vi "Convert String.vi"(4 "dst byte order":T3(ring), 5 "src channel descriptor":T1 {"buffer offset" format="%d bytes"}, 6 "src byte order":T3(ring), 7 "dst channel descriptor":T1 {"buffer offset" format="%d bytes"}, 8 "error in (no error)":errorcluster, 9 "channel count":u64, 10 "dst buffer in":string, 11 "src buffer in":string) -> (0 "error out":errorcluster, 2 "dst buffer out":string, 3 "src buffer out":string)   [LabVIEW 2017, in "DSF Core.lvlib" / "Buffer Converter.lvclass"]
uses:
  Buffer Converter.lvclass
  Block Descriptor.ctl
  DSF Configuration API/Public/Controls/DSF Data Type.ctl
  Shared/VIs/Sizeof.vi
  DSF Core.lvlib
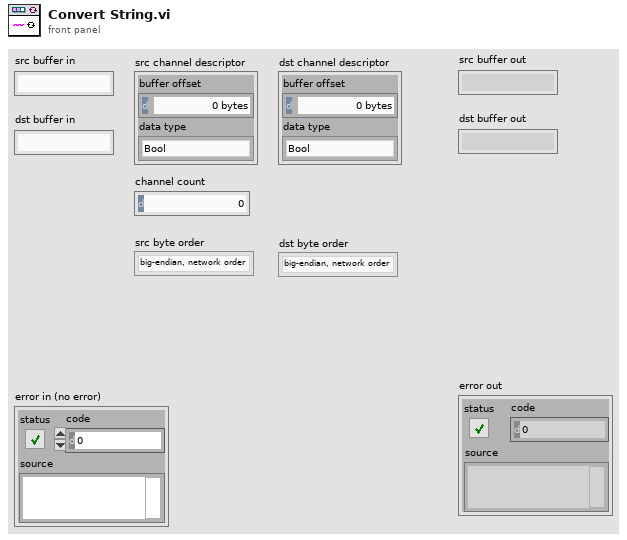
[diagram p1: front panel]
types:
  T1 = typedef "DSF Core.lvlib/Buffer Converter.lvclass/Block Descriptor.ctl" = cluster{"buffer offset":u64, "data type":T2}
  T2 = typedef "DSF Core.lvlib/DSF Data Type.ctl" = enum8{"Bool", "SGL", "DBL", "I8", "I16", "I32", "I64", "U8", "U16", "U32", "U64"}
  T3 = enum16{"big-endian, network order", "native, host order", "little-endian"}
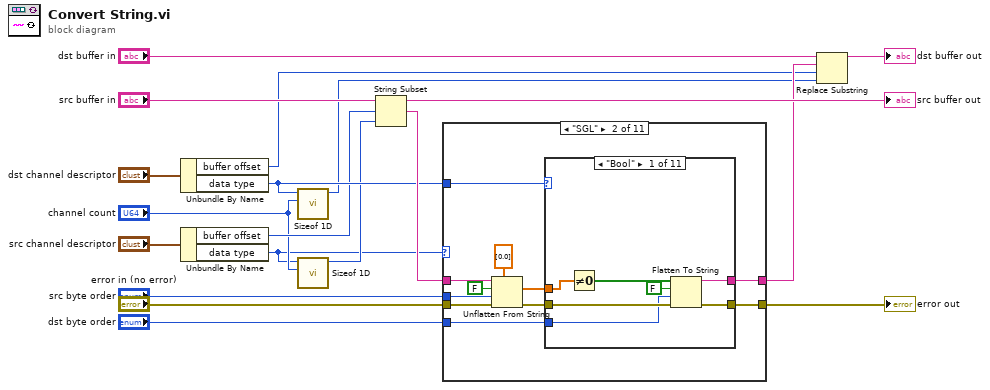
[diagram p0: block diagram]
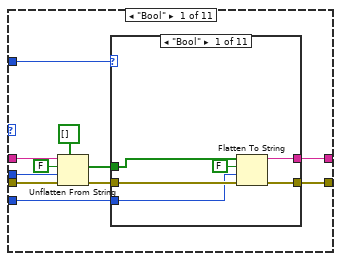
[diagram p2: hidden frame]
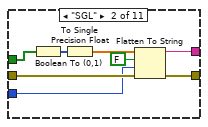
[diagram p3: hidden frame]
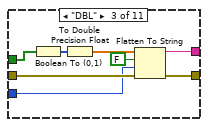
[diagram p4: hidden frame]
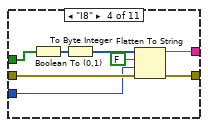
[diagram p5: hidden frame]
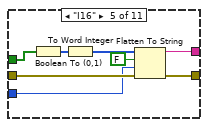
[diagram p6: hidden frame]
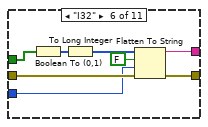
[diagram p7: hidden frame]
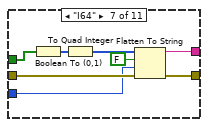
[diagram p8: hidden frame]
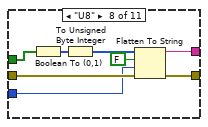
[diagram p9: hidden frame]
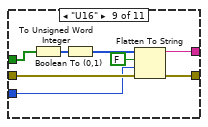
[diagram p10: hidden frame]
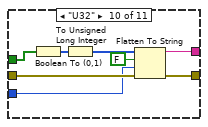
[diagram p11: hidden frame]
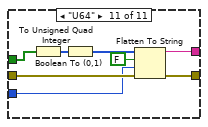
[diagram p12: hidden frame]
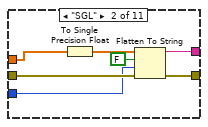
[diagram p13: hidden frame]
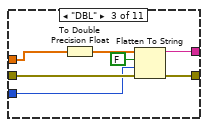
[diagram p14: hidden frame]
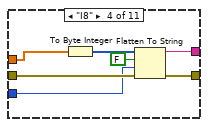
[diagram p15: hidden frame]
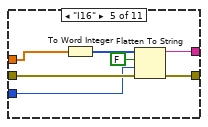
[diagram p16: hidden frame]
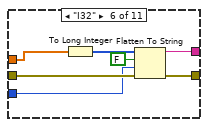
[diagram p17: hidden frame]
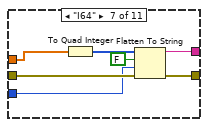
[diagram p18: hidden frame]
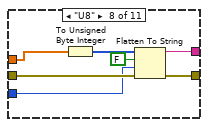
[diagram p19: hidden frame]
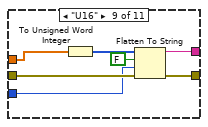
[diagram p20: hidden frame]
diagram:
  n1 = Unbundle By Name("dst channel descriptor") -> ("buffer offset"=w1:u64, "data type"=w10:T2)
  n2 = Unbundle By Name("src channel descriptor") -> ("buffer offset"=w9:u64, "data type"=w4:T2)
  n3 = call "Sizeof 1D.vi"("count"="channel count", "data type"=w10) -> ("size in bytes"=w2:u64)  [unwired: 9 in]
  n4 = call "Sizeof 1D.vi"("count"="channel count", "data type"=w4) -> ("size in bytes"=w8:u64)  [unwired: 9 in]
  n5 = String Subset(string="src buffer in", offset (0)=w9, length (rest)=w8) -> (substring=w11:string)
  n6 = case shown="\"SGL\"" w4 {
    tunnel: w11 -> [w27 w124 w212 w300 w388 w476 w564 w652 w740 w828 w916]
    tunnel: "error in (no error)" -> [w26 w123 w211 w299 w387 w475 w563 w651 w739 w827 w915]
    tunnel: w10 -> [w25 w122 w210 w298 w386 w474 w562 w650 w738 w826 w914]
    tunnel: [w22 w119 w207 w295 w383 w471 w559 w647 w735 w823 w911] -> w16
    tunnel: [w21 w118 w206 w294 w382 w470 w558 w646 w734 w822 w910] -> w3
    tunnel: "src byte order" -> [w20 w117 w205 w293 w381 w469 w557 w645 w733 w821 w909]
    tunnel: "dst byte order" -> [w19 w116 w204 w292 w380 w468 w556 w644 w732 w820 w908]
    frame "Bool" {
      n7 = Unflatten From String(type=bool[] [], binary string=w27, data includes array or string size? (T)=FALSE, byte order (0:big-endian, network order)=w20, error in (no error)=w26) -> (value=w24:bool[], error out=w23:errorcluster)  [unwired: 1 out]
      n8 = case shown="\"Bool\"" w25 {
        tunnel: w24 -> [w35 w43 w51 w59 w67 w75 w83 w91 w99 w107 w115]
        tunnel: w23 -> [w34 w42 w50 w58 w66 w74 w82 w90 w98 w106 w114]
        tunnel: [w33 w41 w49 w57 w65 w73 w81 w89 w97 w105 w113] -> w22
        tunnel: [w32 w40 w48 w56 w64 w72 w80 w88 w96 w104 w112] -> w21
        tunnel: w19 -> [w31 w39 w47 w55 w63 w71 w79 w87 w95 w103 w111]
        frame "Bool" {
          n9 = Flatten To String(anything=w35, prepend array or string size? (T)=FALSE, byte order (0:big-endian, network order)=w31, error in (no error)=w34) -> (data string=w32:string, error out=w33:errorcluster)  [unwired: 1 out]
        }
        frame "SGL" {
          n10 = Boolean To (0,1)(Boolean=w43) -> (0, 1=w36:i16[])
          n11 = To Single Precision Float(number=w36) -> (single precision float=w37:sgl[])
          n12 = Flatten To String(anything=w37, prepend array or string size? (T)=FALSE, byte order (0:big-endian, network order)=w39, error in (no error)=w42) -> (data string=w40:string, error out=w41:errorcluster)  [unwired: 1 out]
        }
        frame "DBL" {
          n13 = Boolean To (0,1)(Boolean=w51) -> (0, 1=w44:i16[])
          n14 = To Double Precision Float(number=w44) -> (double precision float=w45:dbl[])
          n15 = Flatten To String(anything=w45, prepend array or string size? (T)=FALSE, byte order (0:big-endian, network order)=w47, error in (no error)=w50) -> (data string=w48:string, error out=w49:errorcluster)  [unwired: 1 out]
        }
        frame "I8" {
          n16 = Boolean To (0,1)(Boolean=w59) -> (0, 1=w52:i16[])
          n17 = To Byte Integer(number=w52) -> (8bit integer=w53:i8[])
          n18 = Flatten To String(anything=w53, prepend array or string size? (T)=FALSE, byte order (0:big-endian, network order)=w55, error in (no error)=w58) -> (data string=w56:string, error out=w57:errorcluster)  [unwired: 1 out]
        }
        frame "I16" {
          n19 = Boolean To (0,1)(Boolean=w67) -> (0, 1=w60:i16[])
          n20 = To Word Integer(number=w60) -> (16bit integer=w61:i16[])
          n21 = Flatten To String(anything=w61, prepend array or string size? (T)=FALSE, byte order (0:big-endian, network order)=w63, error in (no error)=w66) -> (data string=w64:string, error out=w65:errorcluster)  [unwired: 1 out]
        }
        frame "I32" {
          n22 = Boolean To (0,1)(Boolean=w75) -> (0, 1=w68:i16[])
          n23 = To Long Integer(number=w68) -> (32bit integer=w69:i32[])
          n24 = Flatten To String(anything=w69, prepend array or string size? (T)=FALSE, byte order (0:big-endian, network order)=w71, error in (no error)=w74) -> (data string=w72:string, error out=w73:errorcluster)  [unwired: 1 out]
        }
        frame "I64" {
          n25 = Boolean To (0,1)(Boolean=w83) -> (0, 1=w76:i16[])
          n26 = To Quad Integer(1:w76) -> (0:w77:i64[])
          n27 = Flatten To String(anything=w77, prepend array or string size? (T)=FALSE, byte order (0:big-endian, network order)=w79, error in (no error)=w82) -> (data string=w80:string, error out=w81:errorcluster)  [unwired: 1 out]
        }
        frame "U8" {
          n28 = Boolean To (0,1)(Boolean=w91) -> (0, 1=w84:i16[])
          n29 = To Unsigned Byte Integer(number=w84) -> (unsigned 8bit integer=w85:u8[])
          n30 = Flatten To String(anything=w85, prepend array or string size? (T)=FALSE, byte order (0:big-endian, network order)=w87, error in (no error)=w90) -> (data string=w88:string, error out=w89:errorcluster)  [unwired: 1 out]
        }
        frame "U16" {
          n31 = Boolean To (0,1)(Boolean=w99) -> (0, 1=w92:i16[])
          n32 = To Unsigned Word Integer(number=w92) -> (unsigned 16bit integer=w93:u16[])
          n33 = Flatten To String(anything=w93, prepend array or string size? (T)=FALSE, byte order (0:big-endian, network order)=w95, error in (no error)=w98) -> (data string=w96:string, error out=w97:errorcluster)  [unwired: 1 out]
        }
        frame "U32" {
          n34 = Boolean To (0,1)(Boolean=w107) -> (0, 1=w100:i16[])
          n35 = To Unsigned Long Integer(number=w100) -> (unsigned 32bit integer=w101:u32[])
          n36 = Flatten To String(anything=w101, prepend array or string size? (T)=FALSE, byte order (0:big-endian, network order)=w103, error in (no error)=w106) -> (data string=w104:string, error out=w105:errorcluster)  [unwired: 1 out]
        }
        frame "U64" {
          n37 = Boolean To (0,1)(Boolean=w115) -> (0, 1=w108:i16[])
          n38 = To Unsigned Quad Integer(1:w108) -> (0:w109:u64[])
          n39 = Flatten To String(anything=w109, prepend array or string size? (T)=FALSE, byte order (0:big-endian, network order)=w111, error in (no error)=w114) -> (data string=w112:string, error out=w113:errorcluster)  [unwired: 1 out]
        }
      }
    }
    frame "SGL" {
      n40 = Unflatten From String(type=sgl[] [0.0], binary string=w124, data includes array or string size? (T)=FALSE, byte order (0:big-endian, network order)=w117, error in (no error)=w123) -> (value=w121:sgl[], error out=w120:errorcluster)  [unwired: 1 out]
      n41 = case shown="\"Bool\"" w122 {
        tunnel: w121 -> [w128 w135 w142 w149 w156 w163 w170 w177 w184 w191 w198]
        tunnel: w120 -> [w133 w140 w147 w154 w161 w168 w175 w182 w189 w196 w203]
        tunnel: [w132 w139 w146 w153 w160 w167 w174 w181 w188 w195 w202] -> w119
        tunnel: [w131 w138 w145 w152 w159 w166 w173 w180 w187 w194 w201] -> w118
        tunnel: w116 -> [w130 w137 w144 w151 w158 w165 w172 w179 w186 w193 w200]
        frame "Bool" {
          n42 = Not Equal To 0?(x=w128) -> (x != 0?=w127:bool[])
          n43 = Flatten To String(anything=w127, prepend array or string size? (T)=FALSE, byte order (0:big-endian, network order)=w130, error in (no error)=w133) -> (data string=w131:string, error out=w132:errorcluster)  [unwired: 1 out]
        }
        frame "SGL" {
          n44 = To Single Precision Float(number=w135) -> (single precision float=w134:sgl[])
          n45 = Flatten To String(anything=w134, prepend array or string size? (T)=FALSE, byte order (0:big-endian, network order)=w137, error in (no error)=w140) -> (data string=w138:string, error out=w139:errorcluster)  [unwired: 1 out]
        }
        frame "DBL" {
          n46 = To Double Precision Float(number=w142) -> (double precision float=w141:dbl[])
          n47 = Flatten To String(anything=w141, prepend array or string size? (T)=FALSE, byte order (0:big-endian, network order)=w144, error in (no error)=w147) -> (data string=w145:string, error out=w146:errorcluster)  [unwired: 1 out]
        }
        frame "I8" {
          n48 = To Byte Integer(number=w149) -> (8bit integer=w148:i8[])
          n49 = Flatten To String(anything=w148, prepend array or string size? (T)=FALSE, byte order (0:big-endian, network order)=w151, error in (no error)=w154) -> (data string=w152:string, error out=w153:errorcluster)  [unwired: 1 out]
        }
        frame "I16" {
          n50 = To Word Integer(number=w156) -> (16bit integer=w155:i16[])
          n51 = Flatten To String(anything=w155, prepend array or string size? (T)=FALSE, byte order (0:big-endian, network order)=w158, error in (no error)=w161) -> (data string=w159:string, error out=w160:errorcluster)  [unwired: 1 out]
        }
        frame "I32" {
          n52 = To Long Integer(number=w163) -> (32bit integer=w162:i32[])
          n53 = Flatten To String(anything=w162, prepend array or string size? (T)=FALSE, byte order (0:big-endian, network order)=w165, error in (no error)=w168) -> (data string=w166:string, error out=w167:errorcluster)  [unwired: 1 out]
        }
        frame "I64" {
          n54 = To Quad Integer(1:w170) -> (0:w169:i64[])
          n55 = Flatten To String(anything=w169, prepend array or string size? (T)=FALSE, byte order (0:big-endian, network order)=w172, error in (no error)=w175) -> (data string=w173:string, error out=w174:errorcluster)  [unwired: 1 out]
        }
        frame "U8" {
          n56 = To Unsigned Byte Integer(number=w177) -> (unsigned 8bit integer=w176:u8[])
          n57 = Flatten To String(anything=w176, prepend array or string size? (T)=FALSE, byte order (0:big-endian, network order)=w179, error in (no error)=w182) -> (data string=w180:string, error out=w181:errorcluster)  [unwired: 1 out]
        }
        frame "U16" {
          n58 = To Unsigned Word Integer(number=w184) -> (unsigned 16bit integer=w183:u16[])
          n59 = Flatten To String(anything=w183, prepend array or string size? (T)=FALSE, byte order (0:big-endian, network order)=w186, error in (no error)=w189) -> (data string=w187:string, error out=w188:errorcluster)  [unwired: 1 out]
        }
        frame "U32" {
          n60 = To Unsigned Long Integer(number=w191) -> (unsigned 32bit integer=w190:u32[])
          n61 = Flatten To String(anything=w190, prepend array or string size? (T)=FALSE, byte order (0:big-endian, network order)=w193, error in (no error)=w196) -> (data string=w194:string, error out=w195:errorcluster)  [unwired: 1 out]
        }
        frame "U64" {
          n62 = To Unsigned Quad Integer(1:w198) -> (0:w197:u64[])
          n63 = Flatten To String(anything=w197, prepend array or string size? (T)=FALSE, byte order (0:big-endian, network order)=w200, error in (no error)=w203) -> (data string=w201:string, error out=w202:errorcluster)  [unwired: 1 out]
        }
      }
    }
    frame "DBL" {
      n64 = Unflatten From String(type=dbl[] [0.0], binary string=w212, data includes array or string size? (T)=FALSE, byte order (0:big-endian, network order)=w205, error in (no error)=w211) -> (value=w209:dbl[], error out=w208:errorcluster)  [unwired: 1 out]
      n65 = case shown="\"I8\"" w210 {
        tunnel: w209 -> [w216 w223 w230 w237 w244 w251 w258 w265 w272 w279 w286]
        tunnel: w208 -> [w221 w228 w235 w242 w249 w256 w263 w270 w277 w284 w291]
        tunnel: [w220 w227 w234 w241 w248 w255 w262 w269 w276 w283 w290] -> w207
        tunnel: [w219 w226 w233 w240 w247 w254 w261 w268 w275 w282 w289] -> w206
        tunnel: w204 -> [w218 w225 w232 w239 w246 w253 w260 w267 w274 w281 w288]
        frame "Bool" {
          n66 = Not Equal To 0?(x=w216) -> (x != 0?=w215:bool[])
          n67 = Flatten To String(anything=w215, prepend array or string size? (T)=FALSE, byte order (0:big-endian, network order)=w218, error in (no error)=w221) -> (data string=w219:string, error out=w220:errorcluster)  [unwired: 1 out]
        }
        frame "SGL" {
          n68 = To Single Precision Float(number=w223) -> (single precision float=w222:sgl[])
          n69 = Flatten To String(anything=w222, prepend array or string size? (T)=FALSE, byte order (0:big-endian, network order)=w225, error in (no error)=w228) -> (data string=w226:string, error out=w227:errorcluster)  [unwired: 1 out]
        }
        frame "DBL" {
          n70 = To Double Precision Float(number=w230) -> (double precision float=w229:dbl[])
          n71 = Flatten To String(anything=w229, prepend array or string size? (T)=FALSE, byte order (0:big-endian, network order)=w232, error in (no error)=w235) -> (data string=w233:string, error out=w234:errorcluster)  [unwired: 1 out]
        }
        frame "I8" {
          n72 = To Byte Integer(number=w237) -> (8bit integer=w236:i8[])
          n73 = Flatten To String(anything=w236, prepend array or string size? (T)=FALSE, byte order (0:big-endian, network order)=w239, error in (no error)=w242) -> (data string=w240:string, error out=w241:errorcluster)  [unwired: 1 out]
        }
        frame "I16" {
          n74 = To Word Integer(number=w244) -> (16bit integer=w243:i16[])
          n75 = Flatten To String(anything=w243, prepend array or string size? (T)=FALSE, byte order (0:big-endian, network order)=w246, error in (no error)=w249) -> (data string=w247:string, error out=w248:errorcluster)  [unwired: 1 out]
        }
        frame "I32" {
          n76 = To Long Integer(number=w251) -> (32bit integer=w250:i32[])
          n77 = Flatten To String(anything=w250, prepend array or string size? (T)=FALSE, byte order (0:big-endian, network order)=w253, error in (no error)=w256) -> (data string=w254:string, error out=w255:errorcluster)  [unwired: 1 out]
        }
        frame "I64" {
          n78 = To Quad Integer(1:w258) -> (0:w257:i64[])
          n79 = Flatten To String(anything=w257, prepend array or string size? (T)=FALSE, byte order (0:big-endian, network order)=w260, error in (no error)=w263) -> (data string=w261:string, error out=w262:errorcluster)  [unwired: 1 out]
        }
        frame "U8" {
          n80 = To Unsigned Byte Integer(number=w265) -> (unsigned 8bit integer=w264:u8[])
          n81 = Flatten To String(anything=w264, prepend array or string size? (T)=FALSE, byte order (0:big-endian, network order)=w267, error in (no error)=w270) -> (data string=w268:string, error out=w269:errorcluster)  [unwired: 1 out]
        }
        frame "U16" {
          n82 = To Unsigned Word Integer(number=w272) -> (unsigned 16bit integer=w271:u16[])
          n83 = Flatten To String(anything=w271, prepend array or string size? (T)=FALSE, byte order (0:big-endian, network order)=w274, error in (no error)=w277) -> (data string=w275:string, error out=w276:errorcluster)  [unwired: 1 out]
        }
        frame "U32" {
          n84 = To Unsigned Long Integer(number=w279) -> (unsigned 32bit integer=w278:u32[])
          n85 = Flatten To String(anything=w278, prepend array or string size? (T)=FALSE, byte order (0:big-endian, network order)=w281, error in (no error)=w284) -> (data string=w282:string, error out=w283:errorcluster)  [unwired: 1 out]
        }
        frame "U64" {
          n86 = To Unsigned Quad Integer(1:w286) -> (0:w285:u64[])
          n87 = Flatten To String(anything=w285, prepend array or string size? (T)=FALSE, byte order (0:big-endian, network order)=w288, error in (no error)=w291) -> (data string=w289:string, error out=w290:errorcluster)  [unwired: 1 out]
        }
      }
    }
    frame "I8" {
      n88 = Unflatten From String(type=i8[] [0], binary string=w300, data includes array or string size? (T)=FALSE, byte order (0:big-endian, network order)=w293, error in (no error)=w299) -> (value=w297:i8[], error out=w296:errorcluster)  [unwired: 1 out]
      n89 = case shown="\"Bool\"" w298 {
        tunnel: w297 -> [w304 w311 w318 w325 w332 w339 w346 w353 w360 w367 w374]
        tunnel: w296 -> [w309 w316 w323 w330 w337 w344 w351 w358 w365 w372 w379]
        tunnel: [w308 w315 w322 w329 w336 w343 w350 w357 w364 w371 w378] -> w295
        tunnel: [w307 w314 w321 w328 w335 w342 w349 w356 w363 w370 w377] -> w294
        tunnel: w292 -> [w306 w313 w320 w327 w334 w341 w348 w355 w362 w369 w376]
        frame "Bool" {
          n90 = Not Equal To 0?(x=w304) -> (x != 0?=w303:bool[])
          n91 = Flatten To String(anything=w303, prepend array or string size? (T)=FALSE, byte order (0:big-endian, network order)=w306, error in (no error)=w309) -> (data string=w307:string, error out=w308:errorcluster)  [unwired: 1 out]
        }
        frame "SGL" {
          n92 = To Single Precision Float(number=w311) -> (single precision float=w310:sgl[])
          n93 = Flatten To String(anything=w310, prepend array or string size? (T)=FALSE, byte order (0:big-endian, network order)=w313, error in (no error)=w316) -> (data string=w314:string, error out=w315:errorcluster)  [unwired: 1 out]
        }
        frame "DBL" {
          n94 = To Double Precision Float(number=w318) -> (double precision float=w317:dbl[])
          n95 = Flatten To String(anything=w317, prepend array or string size? (T)=FALSE, byte order (0:big-endian, network order)=w320, error in (no error)=w323) -> (data string=w321:string, error out=w322:errorcluster)  [unwired: 1 out]
        }
        frame "I8" {
          n96 = To Byte Integer(number=w325) -> (8bit integer=w324:i8[])
          n97 = Flatten To String(anything=w324, prepend array or string size? (T)=FALSE, byte order (0:big-endian, network order)=w327, error in (no error)=w330) -> (data string=w328:string, error out=w329:errorcluster)  [unwired: 1 out]
        }
        frame "I16" {
          n98 = To Word Integer(number=w332) -> (16bit integer=w331:i16[])
          n99 = Flatten To String(anything=w331, prepend array or string size? (T)=FALSE, byte order (0:big-endian, network order)=w334, error in (no error)=w337) -> (data string=w335:string, error out=w336:errorcluster)  [unwired: 1 out]
        }
        frame "I32" {
          n100 = To Long Integer(number=w339) -> (32bit integer=w338:i32[])
          n101 = Flatten To String(anything=w338, prepend array or string size? (T)=FALSE, byte order (0:big-endian, network order)=w341, error in (no error)=w344) -> (data string=w342:string, error out=w343:errorcluster)  [unwired: 1 out]
        }
        frame "I64" {
          n102 = To Quad Integer(1:w346) -> (0:w345:i64[])
          n103 = Flatten To String(anything=w345, prepend array or string size? (T)=FALSE, byte order (0:big-endian, network order)=w348, error in (no error)=w351) -> (data string=w349:string, error out=w350:errorcluster)  [unwired: 1 out]
        }
        frame "U8" {
          n104 = To Unsigned Byte Integer(number=w353) -> (unsigned 8bit integer=w352:u8[])
          n105 = Flatten To String(anything=w352, prepend array or string size? (T)=FALSE, byte order (0:big-endian, network order)=w355, error in (no error)=w358) -> (data string=w356:string, error out=w357:errorcluster)  [unwired: 1 out]
        }
        frame "U16" {
          n106 = To Unsigned Word Integer(number=w360) -> (unsigned 16bit integer=w359:u16[])
          n107 = Flatten To String(anything=w359, prepend array or string size? (T)=FALSE, byte order (0:big-endian, network order)=w362, error in (no error)=w365) -> (data string=w363:string, error out=w364:errorcluster)  [unwired: 1 out]
        }
        frame "U32" {
          n108 = To Unsigned Long Integer(number=w367) -> (unsigned 32bit integer=w366:u32[])
          n109 = Flatten To String(anything=w366, prepend array or string size? (T)=FALSE, byte order (0:big-endian, network order)=w369, error in (no error)=w372) -> (data string=w370:string, error out=w371:errorcluster)  [unwired: 1 out]
        }
        frame "U64" {
          n110 = To Unsigned Quad Integer(1:w374) -> (0:w373:u64[])
          n111 = Flatten To String(anything=w373, prepend array or string size? (T)=FALSE, byte order (0:big-endian, network order)=w376, error in (no error)=w379) -> (data string=w377:string, error out=w378:errorcluster)  [unwired: 1 out]
        }
      }
    }
    frame "I16" {
      n112 = Unflatten From String(type=i16[] [0], binary string=w388, data includes array or string size? (T)=FALSE, byte order (0:big-endian, network order)=w381, error in (no error)=w387) -> (value=w385:i16[], error out=w384:errorcluster)  [unwired: 1 out]
      n113 = case shown="\"Bool\"" w386 {
        tunnel: w385 -> [w392 w399 w406 w413 w420 w427 w434 w441 w448 w455 w462]
        tunnel: w384 -> [w397 w404 w411 w418 w425 w432 w439 w446 w453 w460 w467]
        tunnel: [w396 w403 w410 w417 w424 w431 w438 w445 w452 w459 w466] -> w383
        tunnel: [w395 w402 w409 w416 w423 w430 w437 w444 w451 w458 w465] -> w382
        tunnel: w380 -> [w394 w401 w408 w415 w422 w429 w436 w443 w450 w457 w464]
        frame "Bool" {
          n114 = Not Equal To 0?(x=w392) -> (x != 0?=w391:bool[])
          n115 = Flatten To String(anything=w391, prepend array or string size? (T)=FALSE, byte order (0:big-endian, network order)=w394, error in (no error)=w397) -> (data string=w395:string, error out=w396:errorcluster)  [unwired: 1 out]
        }
        frame "SGL" {
          n116 = To Single Precision Float(number=w399) -> (single precision float=w398:sgl[])
          n117 = Flatten To String(anything=w398, prepend array or string size? (T)=FALSE, byte order (0:big-endian, network order)=w401, error in (no error)=w404) -> (data string=w402:string, error out=w403:errorcluster)  [unwired: 1 out]
        }
        frame "DBL" {
          n118 = To Double Precision Float(number=w406) -> (double precision float=w405:dbl[])
          n119 = Flatten To String(anything=w405, prepend array or string size? (T)=FALSE, byte order (0:big-endian, network order)=w408, error in (no error)=w411) -> (data string=w409:string, error out=w410:errorcluster)  [unwired: 1 out]
        }
        frame "I8" {
          n120 = To Byte Integer(number=w413) -> (8bit integer=w412:i8[])
          n121 = Flatten To String(anything=w412, prepend array or string size? (T)=FALSE, byte order (0:big-endian, network order)=w415, error in (no error)=w418) -> (data string=w416:string, error out=w417:errorcluster)  [unwired: 1 out]
        }
        frame "I16" {
          n122 = To Word Integer(number=w420) -> (16bit integer=w419:i16[])
          n123 = Flatten To String(anything=w419, prepend array or string size? (T)=FALSE, byte order (0:big-endian, network order)=w422, error in (no error)=w425) -> (data string=w423:string, error out=w424:errorcluster)  [unwired: 1 out]
        }
        frame "I32" {
          n124 = To Long Integer(number=w427) -> (32bit integer=w426:i32[])
          n125 = Flatten To String(anything=w426, prepend array or string size? (T)=FALSE, byte order (0:big-endian, network order)=w429, error in (no error)=w432) -> (data string=w430:string, error out=w431:errorcluster)  [unwired: 1 out]
        }
        frame "I64" {
          n126 = To Quad Integer(1:w434) -> (0:w433:i64[])
          n127 = Flatten To String(anything=w433, prepend array or string size? (T)=FALSE, byte order (0:big-endian, network order)=w436, error in (no error)=w439) -> (data string=w437:string, error out=w438:errorcluster)  [unwired: 1 out]
        }
        frame "U8" {
          n128 = To Unsigned Byte Integer(number=w441) -> (unsigned 8bit integer=w440:u8[])
          n129 = Flatten To String(anything=w440, prepend array or string size? (T)=FALSE, byte order (0:big-endian, network order)=w443, error in (no error)=w446) -> (data string=w444:string, error out=w445:errorcluster)  [unwired: 1 out]
        }
        frame "U16" {
          n130 = To Unsigned Word Integer(number=w448) -> (unsigned 16bit integer=w447:u16[])
          n131 = Flatten To String(anything=w447, prepend array or string size? (T)=FALSE, byte order (0:big-endian, network order)=w450, error in (no error)=w453) -> (data string=w451:string, error out=w452:errorcluster)  [unwired: 1 out]
        }
        frame "U32" {
          n132 = To Unsigned Long Integer(number=w455) -> (unsigned 32bit integer=w454:u32[])
          n133 = Flatten To String(anything=w454, prepend array or string size? (T)=FALSE, byte order (0:big-endian, network order)=w457, error in (no error)=w460) -> (data string=w458:string, error out=w459:errorcluster)  [unwired: 1 out]
        }
        frame "U64" {
          n134 = To Unsigned Quad Integer(1:w462) -> (0:w461:u64[])
          n135 = Flatten To String(anything=w461, prepend array or string size? (T)=FALSE, byte order (0:big-endian, network order)=w464, error in (no error)=w467) -> (data string=w465:string, error out=w466:errorcluster)  [unwired: 1 out]
        }
      }
    }
    frame "I32" {
      n136 = Unflatten From String(type=i32[] [0], binary string=w476, data includes array or string size? (T)=FALSE, byte order (0:big-endian, network order)=w469, error in (no error)=w475) -> (value=w473:i32[], error out=w472:errorcluster)  [unwired: 1 out]
      n137 = case shown="\"Bool\"" w474 {
        tunnel: w473 -> [w480 w487 w494 w501 w508 w515 w522 w529 w536 w543 w550]
        tunnel: w472 -> [w485 w492 w499 w506 w513 w520 w527 w534 w541 w548 w555]
        tunnel: [w484 w491 w498 w505 w512 w519 w526 w533 w540 w547 w554] -> w471
        tunnel: [w483 w490 w497 w504 w511 w518 w525 w532 w539 w546 w553] -> w470
        tunnel: w468 -> [w482 w489 w496 w503 w510 w517 w524 w531 w538 w545 w552]
        frame "Bool" {
          n138 = Not Equal To 0?(x=w480) -> (x != 0?=w479:bool[])
          n139 = Flatten To String(anything=w479, prepend array or string size? (T)=FALSE, byte order (0:big-endian, network order)=w482, error in (no error)=w485) -> (data string=w483:string, error out=w484:errorcluster)  [unwired: 1 out]
        }
        frame "SGL" {
          n140 = To Single Precision Float(number=w487) -> (single precision float=w486:sgl[])
          n141 = Flatten To String(anything=w486, prepend array or string size? (T)=FALSE, byte order (0:big-endian, network order)=w489, error in (no error)=w492) -> (data string=w490:string, error out=w491:errorcluster)  [unwired: 1 out]
        }
        frame "DBL" {
          n142 = To Double Precision Float(number=w494) -> (double precision float=w493:dbl[])
          n143 = Flatten To String(anything=w493, prepend array or string size? (T)=FALSE, byte order (0:big-endian, network order)=w496, error in (no error)=w499) -> (data string=w497:string, error out=w498:errorcluster)  [unwired: 1 out]
        }
        frame "I8" {
          n144 = To Byte Integer(number=w501) -> (8bit integer=w500:i8[])
          n145 = Flatten To String(anything=w500, prepend array or string size? (T)=FALSE, byte order (0:big-endian, network order)=w503, error in (no error)=w506) -> (data string=w504:string, error out=w505:errorcluster)  [unwired: 1 out]
        }
        frame "I16" {
          n146 = To Word Integer(number=w508) -> (16bit integer=w507:i16[])
          n147 = Flatten To String(anything=w507, prepend array or string size? (T)=FALSE, byte order (0:big-endian, network order)=w510, error in (no error)=w513) -> (data string=w511:string, error out=w512:errorcluster)  [unwired: 1 out]
        }
        frame "I32" {
          n148 = To Long Integer(number=w515) -> (32bit integer=w514:i32[])
          n149 = Flatten To String(anything=w514, prepend array or string size? (T)=FALSE, byte order (0:big-endian, network order)=w517, error in (no error)=w520) -> (data string=w518:string, error out=w519:errorcluster)  [unwired: 1 out]
        }
        frame "I64" {
          n150 = To Quad Integer(1:w522) -> (0:w521:i64[])
          n151 = Flatten To String(anything=w521, prepend array or string size? (T)=FALSE, byte order (0:big-endian, network order)=w524, error in (no error)=w527) -> (data string=w525:string, error out=w526:errorcluster)  [unwired: 1 out]
        }
        frame "U8" {
          n152 = To Unsigned Byte Integer(number=w529) -> (unsigned 8bit integer=w528:u8[])
          n153 = Flatten To String(anything=w528, prepend array or string size? (T)=FALSE, byte order (0:big-endian, network order)=w531, error in (no error)=w534) -> (data string=w532:string, error out=w533:errorcluster)  [unwired: 1 out]
        }
        frame "U16" {
          n154 = To Unsigned Word Integer(number=w536) -> (unsigned 16bit integer=w535:u16[])
          n155 = Flatten To String(anything=w535, prepend array or string size? (T)=FALSE, byte order (0:big-endian, network order)=w538, error in (no error)=w541) -> (data string=w539:string, error out=w540:errorcluster)  [unwired: 1 out]
        }
        frame "U32" {
          n156 = To Unsigned Long Integer(number=w543) -> (unsigned 32bit integer=w542:u32[])
          n157 = Flatten To String(anything=w542, prepend array or string size? (T)=FALSE, byte order (0:big-endian, network order)=w545, error in (no error)=w548) -> (data string=w546:string, error out=w547:errorcluster)  [unwired: 1 out]
        }
        frame "U64" {
          n158 = To Unsigned Quad Integer(1:w550) -> (0:w549:u64[])
          n159 = Flatten To String(anything=w549, prepend array or string size? (T)=FALSE, byte order (0:big-endian, network order)=w552, error in (no error)=w555) -> (data string=w553:string, error out=w554:errorcluster)  [unwired: 1 out]
        }
      }
    }
    frame "I64" {
      n160 = Unflatten From String(type=i64[] [0], binary string=w564, data includes array or string size? (T)=FALSE, byte order (0:big-endian, network order)=w557, error in (no error)=w563) -> (value=w561:i64[], error out=w560:errorcluster)  [unwired: 1 out]
      n161 = case shown="\"Bool\"" w562 {
        tunnel: w561 -> [w568 w575 w582 w589 w596 w603 w610 w617 w624 w631 w638]
        tunnel: w560 -> [w573 w580 w587 w594 w601 w608 w615 w622 w629 w636 w643]
        tunnel: [w572 w579 w586 w593 w600 w607 w614 w621 w628 w635 w642] -> w559
        tunnel: [w571 w578 w585 w592 w599 w606 w613 w620 w627 w634 w641] -> w558
        tunnel: w556 -> [w570 w577 w584 w591 w598 w605 w612 w619 w626 w633 w640]
        frame "Bool" {
          n162 = Not Equal To 0?(x=w568) -> (x != 0?=w567:bool[])
          n163 = Flatten To String(anything=w567, prepend array or string size? (T)=FALSE, byte order (0:big-endian, network order)=w570, error in (no error)=w573) -> (data string=w571:string, error out=w572:errorcluster)  [unwired: 1 out]
        }
        frame "SGL" {
          n164 = To Single Precision Float(number=w575) -> (single precision float=w574:sgl[])
          n165 = Flatten To String(anything=w574, prepend array or string size? (T)=FALSE, byte order (0:big-endian, network order)=w577, error in (no error)=w580) -> (data string=w578:string, error out=w579:errorcluster)  [unwired: 1 out]
        }
        frame "DBL" {
          n166 = To Double Precision Float(number=w582) -> (double precision float=w581:dbl[])
          n167 = Flatten To String(anything=w581, prepend array or string size? (T)=FALSE, byte order (0:big-endian, network order)=w584, error in (no error)=w587) -> (data string=w585:string, error out=w586:errorcluster)  [unwired: 1 out]
        }
        frame "I8" {
          n168 = To Byte Integer(number=w589) -> (8bit integer=w588:i8[])
          n169 = Flatten To String(anything=w588, prepend array or string size? (T)=FALSE, byte order (0:big-endian, network order)=w591, error in (no error)=w594) -> (data string=w592:string, error out=w593:errorcluster)  [unwired: 1 out]
        }
        frame "I16" {
          n170 = To Word Integer(number=w596) -> (16bit integer=w595:i16[])
          n171 = Flatten To String(anything=w595, prepend array or string size? (T)=FALSE, byte order (0:big-endian, network order)=w598, error in (no error)=w601) -> (data string=w599:string, error out=w600:errorcluster)  [unwired: 1 out]
        }
        frame "I32" {
          n172 = To Long Integer(number=w603) -> (32bit integer=w602:i32[])
          n173 = Flatten To String(anything=w602, prepend array or string size? (T)=FALSE, byte order (0:big-endian, network order)=w605, error in (no error)=w608) -> (data string=w606:string, error out=w607:errorcluster)  [unwired: 1 out]
        }
        frame "I64" {
          n174 = To Quad Integer(1:w610) -> (0:w609:i64[])
          n175 = Flatten To String(anything=w609, prepend array or string size? (T)=FALSE, byte order (0:big-endian, network order)=w612, error in (no error)=w615) -> (data string=w613:string, error out=w614:errorcluster)  [unwired: 1 out]
        }
        frame "U8" {
          n176 = To Unsigned Byte Integer(number=w617) -> (unsigned 8bit integer=w616:u8[])
          n177 = Flatten To String(anything=w616, prepend array or string size? (T)=FALSE, byte order (0:big-endian, network order)=w619, error in (no error)=w622) -> (data string=w620:string, error out=w621:errorcluster)  [unwired: 1 out]
        }
        frame "U16" {
          n178 = To Unsigned Word Integer(number=w624) -> (unsigned 16bit integer=w623:u16[])
          n179 = Flatten To String(anything=w623, prepend array or string size? (T)=FALSE, byte order (0:big-endian, network order)=w626, error in (no error)=w629) -> (data string=w627:string, error out=w628:errorcluster)  [unwired: 1 out]
        }
        frame "U32" {
          n180 = To Unsigned Long Integer(number=w631) -> (unsigned 32bit integer=w630:u32[])
          n181 = Flatten To String(anything=w630, prepend array or string size? (T)=FALSE, byte order (0:big-endian, network order)=w633, error in (no error)=w636) -> (data string=w634:string, error out=w635:errorcluster)  [unwired: 1 out]
        }
        frame "U64" {
          n182 = To Unsigned Quad Integer(1:w638) -> (0:w637:u64[])
          n183 = Flatten To String(anything=w637, prepend array or string size? (T)=FALSE, byte order (0:big-endian, network order)=w640, error in (no error)=w643) -> (data string=w641:string, error out=w642:errorcluster)  [unwired: 1 out]
        }
      }
    }
    frame "U8" {
      n184 = Unflatten From String(type=u8[] [0], binary string=w652, data includes array or string size? (T)=FALSE, byte order (0:big-endian, network order)=w645, error in (no error)=w651) -> (value=w649:u8[], error out=w648:errorcluster)  [unwired: 1 out]
      n185 = case shown="\"Bool\"" w650 {
        tunnel: w649 -> [w656 w663 w670 w677 w684 w691 w698 w705 w712 w719 w726]
        tunnel: w648 -> [w661 w668 w675 w682 w689 w696 w703 w710 w717 w724 w731]
        tunnel: [w660 w667 w674 w681 w688 w695 w702 w709 w716 w723 w730] -> w647
        tunnel: [w659 w666 w673 w680 w687 w694 w701 w708 w715 w722 w729] -> w646
        tunnel: w644 -> [w658 w665 w672 w679 w686 w693 w700 w707 w714 w721 w728]
        frame "Bool" {
          n186 = Not Equal To 0?(x=w656) -> (x != 0?=w655:bool[])
          n187 = Flatten To String(anything=w655, prepend array or string size? (T)=FALSE, byte order (0:big-endian, network order)=w658, error in (no error)=w661) -> (data string=w659:string, error out=w660:errorcluster)  [unwired: 1 out]
        }
        frame "SGL" {
          n188 = To Single Precision Float(number=w663) -> (single precision float=w662:sgl[])
          n189 = Flatten To String(anything=w662, prepend array or string size? (T)=FALSE, byte order (0:big-endian, network order)=w665, error in (no error)=w668) -> (data string=w666:string, error out=w667:errorcluster)  [unwired: 1 out]
        }
        frame "DBL" {
          n190 = To Double Precision Float(number=w670) -> (double precision float=w669:dbl[])
          n191 = Flatten To String(anything=w669, prepend array or string size? (T)=FALSE, byte order (0:big-endian, network order)=w672, error in (no error)=w675) -> (data string=w673:string, error out=w674:errorcluster)  [unwired: 1 out]
        }
        frame "I8" {
          n192 = To Byte Integer(number=w677) -> (8bit integer=w676:i8[])
          n193 = Flatten To String(anything=w676, prepend array or string size? (T)=FALSE, byte order (0:big-endian, network order)=w679, error in (no error)=w682) -> (data string=w680:string, error out=w681:errorcluster)  [unwired: 1 out]
        }
        frame "I16" {
          n194 = To Word Integer(number=w684) -> (16bit integer=w683:i16[])
          n195 = Flatten To String(anything=w683, prepend array or string size? (T)=FALSE, byte order (0:big-endian, network order)=w686, error in (no error)=w689) -> (data string=w687:string, error out=w688:errorcluster)  [unwired: 1 out]
        }
        frame "I32" {
          n196 = To Long Integer(number=w691) -> (32bit integer=w690:i32[])
          n197 = Flatten To String(anything=w690, prepend array or string size? (T)=FALSE, byte order (0:big-endian, network order)=w693, error in (no error)=w696) -> (data string=w694:string, error out=w695:errorcluster)  [unwired: 1 out]
        }
        frame "I64" {
          n198 = To Quad Integer(1:w698) -> (0:w697:i64[])
          n199 = Flatten To String(anything=w697, prepend array or string size? (T)=FALSE, byte order (0:big-endian, network order)=w700, error in (no error)=w703) -> (data string=w701:string, error out=w702:errorcluster)  [unwired: 1 out]
        }
        frame "U8" {
          n200 = To Unsigned Byte Integer(number=w705) -> (unsigned 8bit integer=w704:u8[])
          n201 = Flatten To String(anything=w704, prepend array or string size? (T)=FALSE, byte order (0:big-endian, network order)=w707, error in (no error)=w710) -> (data string=w708:string, error out=w709:errorcluster)  [unwired: 1 out]
        }
        frame "U16" {
          n202 = To Unsigned Word Integer(number=w712) -> (unsigned 16bit integer=w711:u16[])
          n203 = Flatten To String(anything=w711, prepend array or string size? (T)=FALSE, byte order (0:big-endian, network order)=w714, error in (no error)=w717) -> (data string=w715:string, error out=w716:errorcluster)  [unwired: 1 out]
        }
        frame "U32" {
          n204 = To Unsigned Long Integer(number=w719) -> (unsigned 32bit integer=w718:u32[])
          n205 = Flatten To String(anything=w718, prepend array or string size? (T)=FALSE, byte order (0:big-endian, network order)=w721, error in (no error)=w724) -> (data string=w722:string, error out=w723:errorcluster)  [unwired: 1 out]
        }
        frame "U64" {
          n206 = To Unsigned Quad Integer(1:w726) -> (0:w725:u64[])
          n207 = Flatten To String(anything=w725, prepend array or string size? (T)=FALSE, byte order (0:big-endian, network order)=w728, error in (no error)=w731) -> (data string=w729:string, error out=w730:errorcluster)  [unwired: 1 out]
        }
      }
    }
    frame "U16" {
      n208 = Unflatten From String(type=u16[] [0], binary string=w740, data includes array or string size? (T)=FALSE, byte order (0:big-endian, network order)=w733, error in (no error)=w739) -> (value=w737:u16[], error out=w736:errorcluster)  [unwired: 1 out]
      n209 = case shown="\"Bool\"" w738 {
        tunnel: w737 -> [w744 w751 w758 w765 w772 w779 w786 w793 w800 w807 w814]
        tunnel: w736 -> [w749 w756 w763 w770 w777 w784 w791 w798 w805 w812 w819]
        tunnel: [w748 w755 w762 w769 w776 w783 w790 w797 w804 w811 w818] -> w735
        tunnel: [w747 w754 w761 w768 w775 w782 w789 w796 w803 w810 w817] -> w734
        tunnel: w732 -> [w746 w753 w760 w767 w774 w781 w788 w795 w802 w809 w816]
        frame "Bool" {
          n210 = Not Equal To 0?(x=w744) -> (x != 0?=w743:bool[])
          n211 = Flatten To String(anything=w743, prepend array or string size? (T)=FALSE, byte order (0:big-endian, network order)=w746, error in (no error)=w749) -> (data string=w747:string, error out=w748:errorcluster)  [unwired: 1 out]
        }
        frame "SGL" {
          n212 = To Single Precision Float(number=w751) -> (single precision float=w750:sgl[])
          n213 = Flatten To String(anything=w750, prepend array or string size? (T)=FALSE, byte order (0:big-endian, network order)=w753, error in (no error)=w756) -> (data string=w754:string, error out=w755:errorcluster)  [unwired: 1 out]
        }
        frame "DBL" {
          n214 = To Double Precision Float(number=w758) -> (double precision float=w757:dbl[])
          n215 = Flatten To String(anything=w757, prepend array or string size? (T)=FALSE, byte order (0:big-endian, network order)=w760, error in (no error)=w763) -> (data string=w761:string, error out=w762:errorcluster)  [unwired: 1 out]
        }
        frame "I8" {
          n216 = To Byte Integer(number=w765) -> (8bit integer=w764:i8[])
          n217 = Flatten To String(anything=w764, prepend array or string size? (T)=FALSE, byte order (0:big-endian, network order)=w767, error in (no error)=w770) -> (data string=w768:string, error out=w769:errorcluster)  [unwired: 1 out]
        }
        frame "I16" {
          n218 = To Word Integer(number=w772) -> (16bit integer=w771:i16[])
          n219 = Flatten To String(anything=w771, prepend array or string size? (T)=FALSE, byte order (0:big-endian, network order)=w774, error in (no error)=w777) -> (data string=w775:string, error out=w776:errorcluster)  [unwired: 1 out]
        }
        frame "I32" {
          n220 = To Long Integer(number=w779) -> (32bit integer=w778:i32[])
          n221 = Flatten To String(anything=w778, prepend array or string size? (T)=FALSE, byte order (0:big-endian, network order)=w781, error in (no error)=w784) -> (data string=w782:string, error out=w783:errorcluster)  [unwired: 1 out]
        }
        frame "I64" {
          n222 = To Quad Integer(1:w786) -> (0:w785:i64[])
          n223 = Flatten To String(anything=w785, prepend array or string size? (T)=FALSE, byte order (0:big-endian, network order)=w788, error in (no error)=w791) -> (data string=w789:string, error out=w790:errorcluster)  [unwired: 1 out]
        }
        frame "U8" {
          n224 = To Unsigned Byte Integer(number=w793) -> (unsigned 8bit integer=w792:u8[])
          n225 = Flatten To String(anything=w792, prepend array or string size? (T)=FALSE, byte order (0:big-endian, network order)=w795, error in (no error)=w798) -> (data string=w796:string, error out=w797:errorcluster)  [unwired: 1 out]
        }
        frame "U16" {
          n226 = To Unsigned Word Integer(number=w800) -> (unsigned 16bit integer=w799:u16[])
          n227 = Flatten To String(anything=w799, prepend array or string size? (T)=FALSE, byte order (0:big-endian, network order)=w802, error in (no error)=w805) -> (data string=w803:string, error out=w804:errorcluster)  [unwired: 1 out]
        }
        frame "U32" {
          n228 = To Unsigned Long Integer(number=w807) -> (unsigned 32bit integer=w806:u32[])
          n229 = Flatten To String(anything=w806, prepend array or string size? (T)=FALSE, byte order (0:big-endian, network order)=w809, error in (no error)=w812) -> (data string=w810:string, error out=w811:errorcluster)  [unwired: 1 out]
        }
        frame "U64" {
          n230 = To Unsigned Quad Integer(1:w814) -> (0:w813:u64[])
          n231 = Flatten To String(anything=w813, prepend array or string size? (T)=FALSE, byte order (0:big-endian, network order)=w816, error in (no error)=w819) -> (data string=w817:string, error out=w818:errorcluster)  [unwired: 1 out]
        }
      }
    }
    frame "U32" {
      n232 = Unflatten From String(type=u32[] [0], binary string=w828, data includes array or string size? (T)=FALSE, byte order (0:big-endian, network order)=w821, error in (no error)=w827) -> (value=w825:u32[], error out=w824:errorcluster)  [unwired: 1 out]
      n233 = case shown="\"Bool\"" w826 {
        tunnel: w825 -> [w832 w839 w846 w853 w860 w867 w874 w881 w888 w895 w902]
        tunnel: w824 -> [w837 w844 w851 w858 w865 w872 w879 w886 w893 w900 w907]
        tunnel: [w836 w843 w850 w857 w864 w871 w878 w885 w892 w899 w906] -> w823
        tunnel: [w835 w842 w849 w856 w863 w870 w877 w884 w891 w898 w905] -> w822
        tunnel: w820 -> [w834 w841 w848 w855 w862 w869 w876 w883 w890 w897 w904]
        frame "Bool" {
          n234 = Not Equal To 0?(x=w832) -> (x != 0?=w831:bool[])
          n235 = Flatten To String(anything=w831, prepend array or string size? (T)=FALSE, byte order (0:big-endian, network order)=w834, error in (no error)=w837) -> (data string=w835:string, error out=w836:errorcluster)  [unwired: 1 out]
        }
        frame "SGL" {
          n236 = To Single Precision Float(number=w839) -> (single precision float=w838:sgl[])
          n237 = Flatten To String(anything=w838, prepend array or string size? (T)=FALSE, byte order (0:big-endian, network order)=w841, error in (no error)=w844) -> (data string=w842:string, error out=w843:errorcluster)  [unwired: 1 out]
        }
        frame "DBL" {
          n238 = To Double Precision Float(number=w846) -> (double precision float=w845:dbl[])
          n239 = Flatten To String(anything=w845, prepend array or string size? (T)=FALSE, byte order (0:big-endian, network order)=w848, error in (no error)=w851) -> (data string=w849:string, error out=w850:errorcluster)  [unwired: 1 out]
        }
        frame "I8" {
          n240 = To Byte Integer(number=w853) -> (8bit integer=w852:i8[])
          n241 = Flatten To String(anything=w852, prepend array or string size? (T)=FALSE, byte order (0:big-endian, network order)=w855, error in (no error)=w858) -> (data string=w856:string, error out=w857:errorcluster)  [unwired: 1 out]
        }
        frame "I16" {
          n242 = To Word Integer(number=w860) -> (16bit integer=w859:i16[])
          n243 = Flatten To String(anything=w859, prepend array or string size? (T)=FALSE, byte order (0:big-endian, network order)=w862, error in (no error)=w865) -> (data string=w863:string, error out=w864:errorcluster)  [unwired: 1 out]
        }
        frame "I32" {
          n244 = To Long Integer(number=w867) -> (32bit integer=w866:i32[])
          n245 = Flatten To String(anything=w866, prepend array or string size? (T)=FALSE, byte order (0:big-endian, network order)=w869, error in (no error)=w872) -> (data string=w870:string, error out=w871:errorcluster)  [unwired: 1 out]
        }
        frame "I64" {
          n246 = To Quad Integer(1:w874) -> (0:w873:i64[])
          n247 = Flatten To String(anything=w873, prepend array or string size? (T)=FALSE, byte order (0:big-endian, network order)=w876, error in (no error)=w879) -> (data string=w877:string, error out=w878:errorcluster)  [unwired: 1 out]
        }
        frame "U8" {
          n248 = To Unsigned Byte Integer(number=w881) -> (unsigned 8bit integer=w880:u8[])
          n249 = Flatten To String(anything=w880, prepend array or string size? (T)=FALSE, byte order (0:big-endian, network order)=w883, error in (no error)=w886) -> (data string=w884:string, error out=w885:errorcluster)  [unwired: 1 out]
        }
        frame "U16" {
          n250 = To Unsigned Word Integer(number=w888) -> (unsigned 16bit integer=w887:u16[])
          n251 = Flatten To String(anything=w887, prepend array or string size? (T)=FALSE, byte order (0:big-endian, network order)=w890, error in (no error)=w893) -> (data string=w891:string, error out=w892:errorcluster)  [unwired: 1 out]
        }
        frame "U32" {
          n252 = To Unsigned Long Integer(number=w895) -> (unsigned 32bit integer=w894:u32[])
          n253 = Flatten To String(anything=w894, prepend array or string size? (T)=FALSE, byte order (0:big-endian, network order)=w897, error in (no error)=w900) -> (data string=w898:string, error out=w899:errorcluster)  [unwired: 1 out]
        }
        frame "U64" {
          n254 = To Unsigned Quad Integer(1:w902) -> (0:w901:u64[])
          n255 = Flatten To String(anything=w901, prepend array or string size? (T)=FALSE, byte order (0:big-endian, network order)=w904, error in (no error)=w907) -> (data string=w905:string, error out=w906:errorcluster)  [unwired: 1 out]
        }
      }
    }
    frame "U64" {
      n256 = Unflatten From String(type=u64[] [0], binary string=w916, data includes array or string size? (T)=FALSE, byte order (0:big-endian, network order)=w909, error in (no error)=w915) -> (value=w913:u64[], error out=w912:errorcluster)  [unwired: 1 out]
      n257 = case shown="\"Bool\"" w914 {
        tunnel: w913 -> [w920 w927 w934 w941 w948 w955 w962 w969 w976 w983 w990]
        tunnel: w912 -> [w925 w932 w939 w946 w953 w960 w967 w974 w981 w988 w995]
        tunnel: [w924 w931 w938 w945 w952 w959 w966 w973 w980 w987 w994] -> w911
        tunnel: [w923 w930 w937 w944 w951 w958 w965 w972 w979 w986 w993] -> w910
        tunnel: w908 -> [w922 w929 w936 w943 w950 w957 w964 w971 w978 w985 w992]
        frame "Bool" {
          n258 = Not Equal To 0?(x=w920) -> (x != 0?=w919:bool[])
          n259 = Flatten To String(anything=w919, prepend array or string size? (T)=FALSE, byte order (0:big-endian, network order)=w922, error in (no error)=w925) -> (data string=w923:string, error out=w924:errorcluster)  [unwired: 1 out]
        }
        frame "SGL" {
          n260 = To Single Precision Float(number=w927) -> (single precision float=w926:sgl[])
          n261 = Flatten To String(anything=w926, prepend array or string size? (T)=FALSE, byte order (0:big-endian, network order)=w929, error in (no error)=w932) -> (data string=w930:string, error out=w931:errorcluster)  [unwired: 1 out]
        }
        frame "DBL" {
          n262 = To Double Precision Float(number=w934) -> (double precision float=w933:dbl[])
          n263 = Flatten To String(anything=w933, prepend array or string size? (T)=FALSE, byte order (0:big-endian, network order)=w936, error in (no error)=w939) -> (data string=w937:string, error out=w938:errorcluster)  [unwired: 1 out]
        }
        frame "I8" {
          n264 = To Byte Integer(number=w941) -> (8bit integer=w940:i8[])
          n265 = Flatten To String(anything=w940, prepend array or string size? (T)=FALSE, byte order (0:big-endian, network order)=w943, error in (no error)=w946) -> (data string=w944:string, error out=w945:errorcluster)  [unwired: 1 out]
        }
        frame "I16" {
          n266 = To Word Integer(number=w948) -> (16bit integer=w947:i16[])
          n267 = Flatten To String(anything=w947, prepend array or string size? (T)=FALSE, byte order (0:big-endian, network order)=w950, error in (no error)=w953) -> (data string=w951:string, error out=w952:errorcluster)  [unwired: 1 out]
        }
        frame "I32" {
          n268 = To Long Integer(number=w955) -> (32bit integer=w954:i32[])
          n269 = Flatten To String(anything=w954, prepend array or string size? (T)=FALSE, byte order (0:big-endian, network order)=w957, error in (no error)=w960) -> (data string=w958:string, error out=w959:errorcluster)  [unwired: 1 out]
        }
        frame "I64" {
          n270 = To Quad Integer(1:w962) -> (0:w961:i64[])
          n271 = Flatten To String(anything=w961, prepend array or string size? (T)=FALSE, byte order (0:big-endian, network order)=w964, error in (no error)=w967) -> (data string=w965:string, error out=w966:errorcluster)  [unwired: 1 out]
        }
        frame "U8" {
          n272 = To Unsigned Byte Integer(number=w969) -> (unsigned 8bit integer=w968:u8[])
          n273 = Flatten To String(anything=w968, prepend array or string size? (T)=FALSE, byte order (0:big-endian, network order)=w971, error in (no error)=w974) -> (data string=w972:string, error out=w973:errorcluster)  [unwired: 1 out]
        }
        frame "U16" {
          n274 = To Unsigned Word Integer(number=w976) -> (unsigned 16bit integer=w975:u16[])
          n275 = Flatten To String(anything=w975, prepend array or string size? (T)=FALSE, byte order (0:big-endian, network order)=w978, error in (no error)=w981) -> (data string=w979:string, error out=w980:errorcluster)  [unwired: 1 out]
        }
        frame "U32" {
          n276 = To Unsigned Long Integer(number=w983) -> (unsigned 32bit integer=w982:u32[])
          n277 = Flatten To String(anything=w982, prepend array or string size? (T)=FALSE, byte order (0:big-endian, network order)=w985, error in (no error)=w988) -> (data string=w986:string, error out=w987:errorcluster)  [unwired: 1 out]
        }
        frame "U64" {
          n278 = To Unsigned Quad Integer(1:w990) -> (0:w989:u64[])
          n279 = Flatten To String(anything=w989, prepend array or string size? (T)=FALSE, byte order (0:big-endian, network order)=w992, error in (no error)=w995) -> (data string=w993:string, error out=w994:errorcluster)  [unwired: 1 out]
        }
      }
    }
  }
  "error out" <- w16
  n280 = Replace Substring(2:w2, 3:w1, 4:w3, 5:"dst buffer in") -> (1:→"dst buffer out":string)  [unwired: 1 out]
  "src buffer out" <- "src buffer in"
